vi "art_pass.vi"(6 "Projection Pixels":T2(array[cluster]), 8 "Ctl Refnum":refnum<vi>, 9 "Projections":T1[](array[typedef]), 10 "image width":i32, 11 "Output in":sgl[](array[numeric])) -> (1 "ART output":sgl[](array[numeric]), 2 "Output out":sgl[](array[numeric]), 3 "Projection":i32)   [LabVIEW 2013]
uses:
  bp_work_unit.ctl
  imagereconstruction/x64/Debug/labviewdll.dll
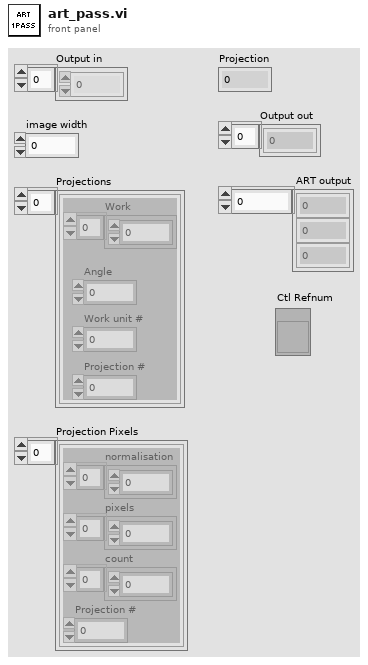
[diagram p1: front panel]
types:
  T1 = typedef "bp_work_unit.ctl" = cluster{"Work":u8[], "Angle":dbl, "Work unit #":i32, "Projection #":i32}
  T2 = cluster{"normalisation":i32[], "pixels":i32[], "count":i32[], "Projection #":i32}[]
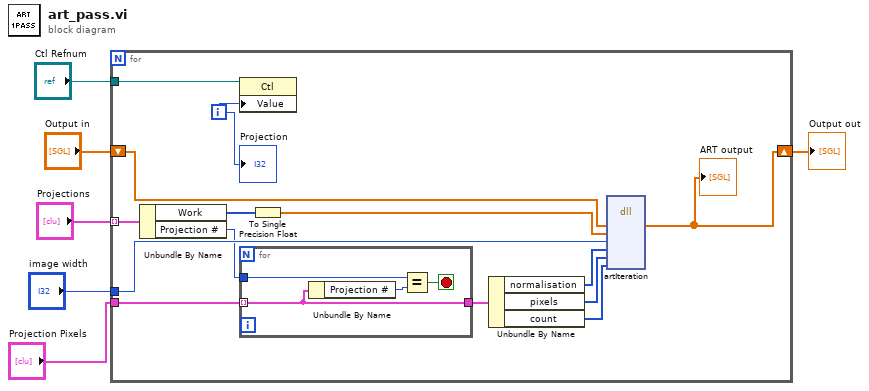
[diagram p0: block diagram]
diagram:
  n1 = for {
    shift-right: [w7] -> w3
    shift-left: "Output in" -> [w20]
    tunnel: "image width" -> [w19]
    tunnel: "Projections" -> [w18] mode=indexing
    tunnel: "Projection Pixels" -> [w17]
    tunnel: "Ctl Refnum" -> [w9]
    i -> [w8]
    n2 = Unbundle By Name(w18) -> ("Work"=w11:u8[], "Projection #"=w16:i32)
    n3 = property class="Ctl"(reference=w9, "Value"=w8) -> ()  [unwired: 1 in, 2 out]
    n4 = for {
      tunnel: w17 -> [w21] mode=indexing
      tunnel: w16 -> [w23]
      tunnel: [w21] -> w15
      stop <- w22 stop-if-true
      n5 = Unbundle By Name(w21) -> ("Projection #"=w24:i32)
      n6 = Equal?(x=w23, y=w24) -> (x = y?=w22:bool)
    }
    n7 = To Single Precision Float(number=w11) -> (single precision float=w10:sgl[])
    n8 = Unbundle By Name(w15) -> ("normalisation"=w14:i32[], "pixels"=w13:i32[], "count"=w12:i32[])
    n9 = dll-call lib="D:/work/uni/FYP/reconrepo/imagereconstruction/x64/Debug/labviewdll.dll" fn="artIteration"("object"=w20, "actual projection"=w10, "w"=w19, "ray normalisation"=w14, "pixels"=w13, "count"=w12) -> ("object"=w7:sgl[])  [unwired: 9 in, 2 out]
    "ART output" <- w7
    "Projection" <- w8
  }
  "Output out" <- w3
